vi "Simulated1.vi"() -> ()   [LabVIEW 2011]
doc: "This VI demonstrates how to control a simulated Robotics Starter Kit 1.0 robot. With a few modifications, you can deploy this VI to the Single-Board RIO 9631 on a real robot, and it runs on the real-time controller. For more information about how to modify this VI so you can deploy it to real hardware, refer to the <B>Robotics Module>>Simulating Mobile Robots</B> book on the <B>Contents</B> tab of the LabVIEW Help."
uses:
  <vilib>/Platform/TimedLoop/XDataNode/XDataNode.xnode
  <vilib>/Platform/TimedLoop/XDataNode/nitl_modes.ctl
  <vilib>/Platform/TimedLoop/XDataNode/XDNodeRunTimeDep.lvlib
  <vilib>/Platform/TimedLoop/XDataNode/wakeup.ctl
  <vilib>/Platform/TimedLoop/XDataNode/timing_clust.ctl
  <vilib>/robotics/Starter Kit/1.0/Sim Host Interface/NI_Robotics_Starter Kit Host_Sim_1.0.lvclass
  <vilib>/robotics/Simulator/NI_Robotics_Simulator.lvlib
  <vilib>/Analysis/Matrix/NI_Matrix.lvlib
  <vilib>/robotics/Starter Kit/Host Interface/NI_Robotics_Starter Kit Host.lvclass
  <vilib>/Analysis/Matrix/Numeric/Conversions/Array To Matrix - RA.vi
  <vilib>/Analysis/Matrix/Datatypes/RealMatrix.ctl
panel:
  out "Zigmar":dbl[](array[numeric])
  out "Zigma":dbl[](array[numeric])
  out "Xr-X":dbl[](array[numeric])
  out "Error":T1
  out "XY Graph":cluster{dbl[], dbl[]}(graph)
  in  "Kp W":dbl step=0.01
  in  "Kp VL":dbl step=0.01
  out "Numeric":i32
  in  "Paso":dbl
  in  "Tiempo":dbl
  in  "stop":bool
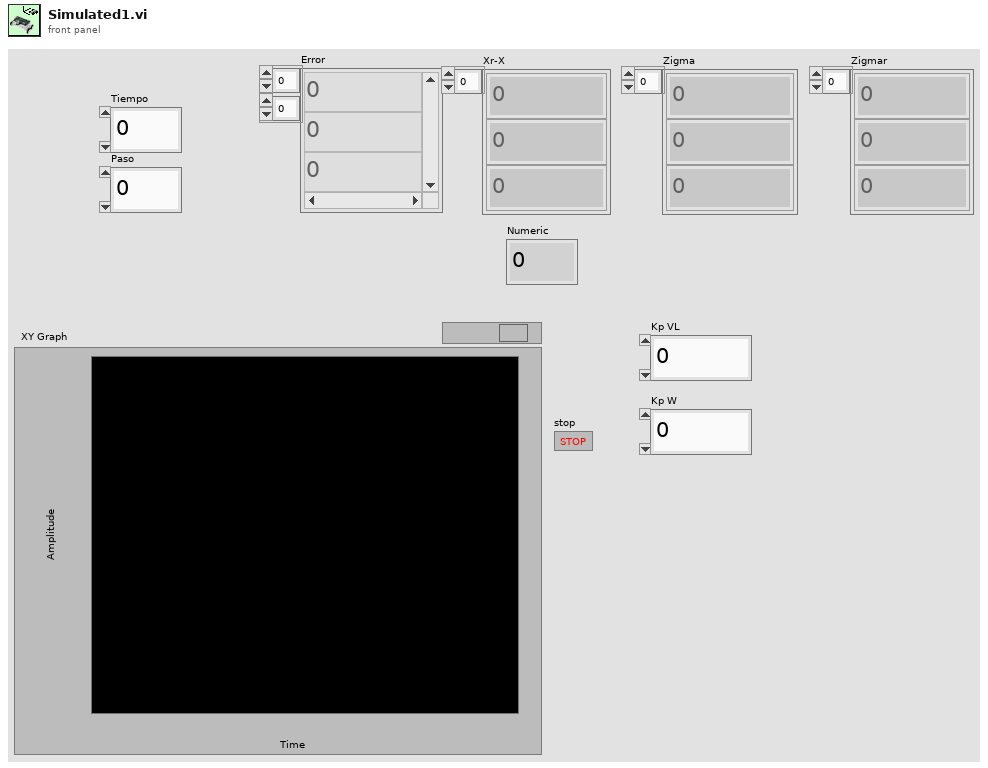
[diagram p1: front panel]
types:
  T1 = typedef "NI_Matrix.lvlib/RealMatrix.ctl" = dbl[][]
  T2 = typedef "XDNodeRunTimeDep.lvlib/timing_clust.ctl" = cluster{"Expected End [f-1]":u64, "Actual End [f-1]":u64, "Finished Late? [f-1]":bool, "Expected End [i-1]":u64, "Actual End [i-1]":u64, "Finished Late? [i-1]":bool, "Expected Start [i]":u64, "Actual Start [i]":u64, "Expected Start [f]":u64, "Actual Start [f]":u64, "Source Name":string, "Structure Name":string, "Period":i64, "Deadline":i64, "Offset":i64, "Start":i64, "Priority":i32, "Timeout":i32, "Mode":T3, "Wakeup Reason":T4, "Error":errorcluster, "Source Type":string, "Secondary Source Type":string, "Global End Time":u64, "Global Start Time":u64, "Frame Duration":u64, "Iteration Duration":u64, "Assigned CPU":i32, "I/O Scan Engine Mode":u32}
  T3 = typedef "XDNodeRunTimeDep.lvlib/nitl_modes.ctl" = enum32{"No Change", "Process missed periods, maintain original phase", "Discard missed periods, maintain original phase", "Process missed periods, ignore original phase", "Discard missed periods, ignore original phase"}
  T4 = typedef "XDNodeRunTimeDep.lvlib/wakeup.ctl" = enum32{"Normal", "Aborted", "Asynchronous wakeup", "Timing source error", "Timed loop error", "Timeout"}
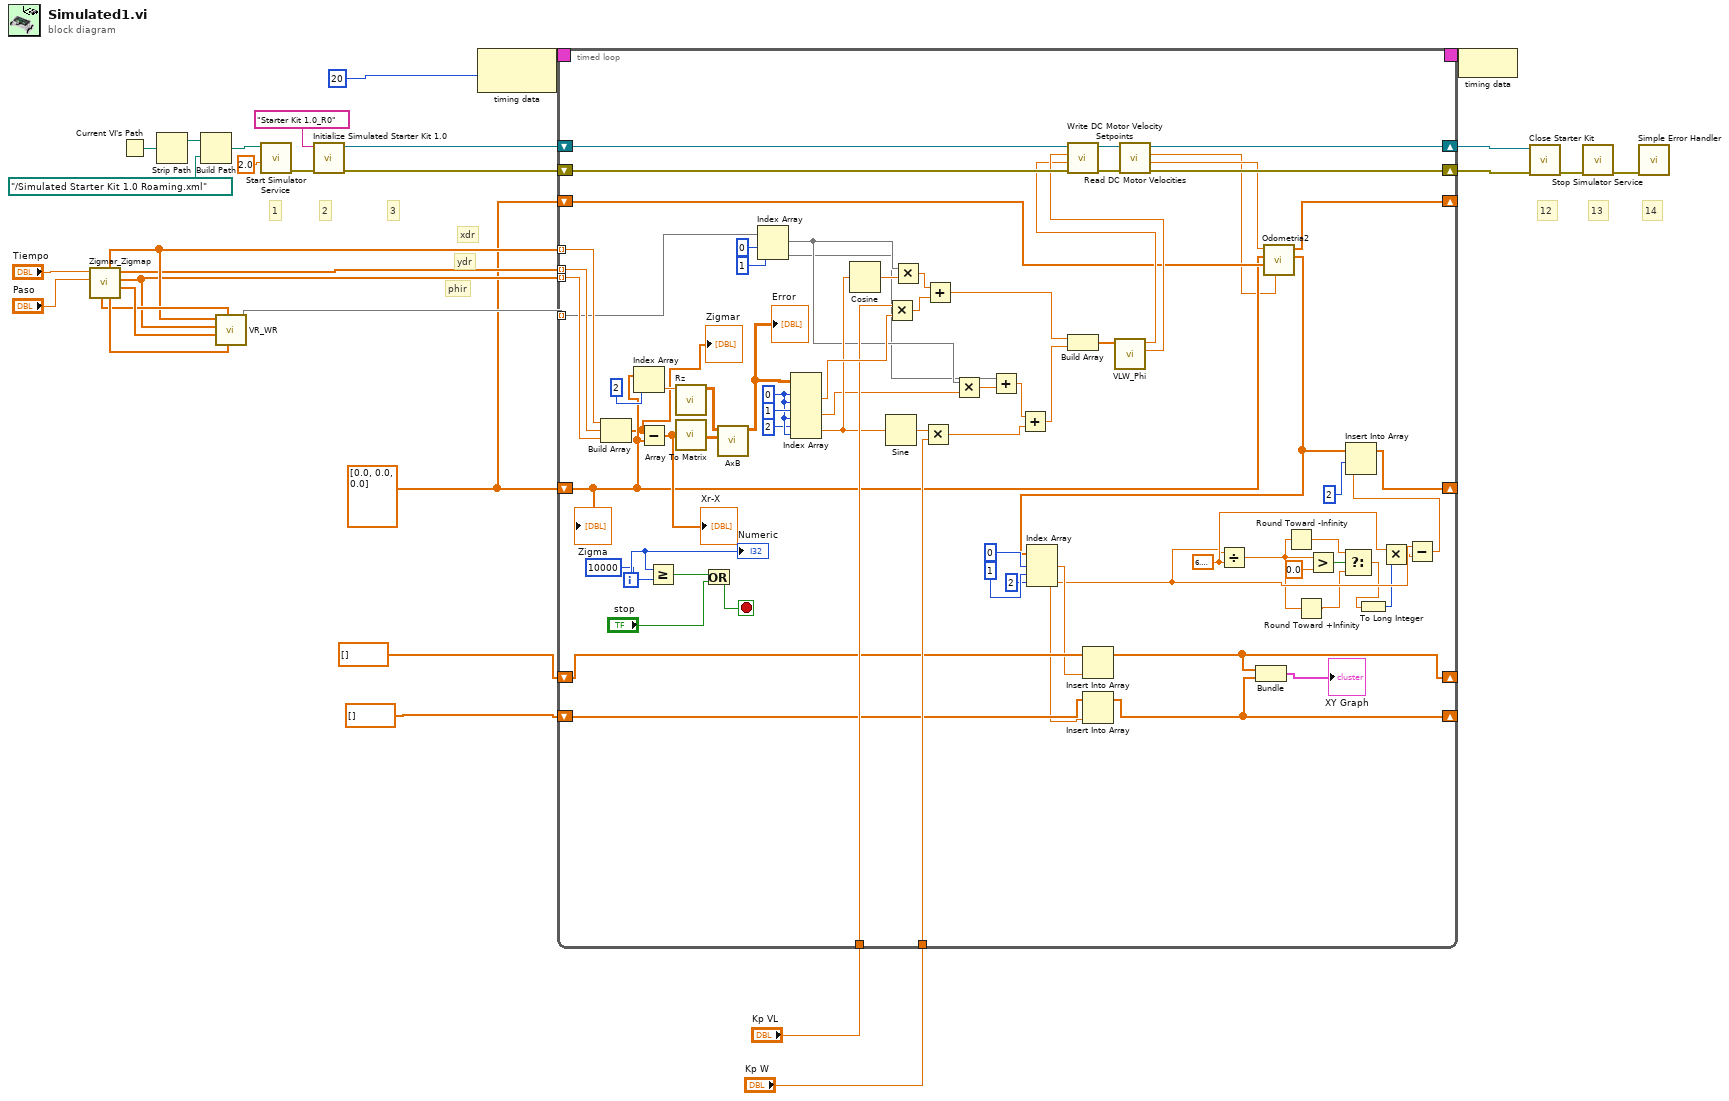
[diagram p0: block diagram]
diagram:
  w3 = dbl[] [0.0, 0.0, 0.0]
  # "phir"
  # "ydr"
  # "xdr"
  # "14"
  # "13"
  # "12"
  # "3"
  # "2"
  # "1"
  n1 = call "Zigmar_Zigmap.vi"("Paso"="Paso", "Tiempo"="Tiempo") -> ("Xdrp"=w11:dbl[], "Phir"=w6:dbl[], "Ydr"=w7:dbl[], "Ydrp"=w12:dbl[], "Xdr"=w8:dbl[], "Phirp"=w10:dbl[])  [unwired: 4 in]
  n2 = Current VI's Path() -> (path=w29:path)
  n3 = Strip Path(path=w29) -> (stripped path=w30:path)  [unwired: 1 out]
  n4 = Build Path(base path=w30, name or relative path=path "../Simulated Starter Kit 1.0 Roaming.xml" ("Simulation Manifest File")) -> (appended path=w20:path)
  n5 = call "VR_WR.vi"("Ydrp"=w12, "Phirp"=w10, "Xdrp"=w11, "Phir"=w6, 11:w8) -> (3:w9)  [unwired: 6 in]
  n6 = call <vilib>:"Start Simulator Service.vi"("step size (ms)"=2.0, "manifest file"=w20) -> ("error out"=w18:errorcluster)  [unwired: 9 in]
  n7 = call <vilib>:"Initialize Simulated Starter Kit 1.0.vi"("error in (no error)"=w18, "robot ID"="Starter Kit 1.0_R0") -> ("error out"=w15:errorcluster, "simulated starter kit host 1.0 out"=w25:refnum<class "NI_Robotics_Starter Kit Host_Sim_1.0.lvclass">)  [unwired: 8 in]
  n8 = node-c288(i64 20 ("Period")) -> (w28:T2)
  n9 = timed-loop {
    shift-right: [w68] -> w24
    shift-left: w25 -> [w70]
    shift-right: [w67] -> w23
    shift-left: w15 -> [w69]
    timing: w28 -> [_]
    timing-out: [_] -> w27
    tunnel: w9 -> [w93] mode=indexing
    tunnel: w8 -> [w105] mode=indexing
    tunnel: w7 -> [w104] mode=indexing
    tunnel: w6 -> [w103] mode=indexing
    shift-right: [w41] -> _
    shift-left: w3 -> [w59]
    tunnel: "Kp VL" -> [w88]
    tunnel: "Kp W" -> [w82]
    shift-right: [w60] -> _
    shift-left: w3 -> [w61]
    shift-right: [w52] -> _
    shift-left: dbl[] [] -> [w58]
    shift-right: [w51] -> _
    shift-left: dbl[] [] -> [w54]
    i -> [w64]
    stop <- w100 stop-if-true
    w44 = 6.283185307179586
    w91 = 0 ("index (row)")
    n10 = Build Array(w105, w104, w103) -> (w46:dbl[])
    "Zigmar" <- w46
    n11 = Index Array(array=w59, index=2) -> (element=w102:dbl)
    n12 = Subtract(x=w46, y=w59) -> (x-y=w97:dbl[])
    "Xr-X" <- w97
    n13 = Greater Or Equal?(x=w64, y=10000 ("x")) -> (x >= y?=w62:bool)
    n14 = call "Rz.vi"("theta"=w102) -> ("RotacionalZ"=w98:T1)  [unwired: 10 in]
    n15 = call-poly <vilib>:"Array To Matrix.vi"("Real 1D Array"=w97) -> ("Real Matrix (Column Vector)"=w96:T1)
    n16 = Or(x=w62, y="stop") -> (x .or. y?=w100:bool)
    n17 = call "AxB.vi"("B"=w96, "A"=w98) -> ("AxB"=w47:T1)  [unwired: 9 in]
    "Error" <- w47
    n18 = Index Array(array=w93, index #1=0 ("index"), index #2=1 ("index")) -> (element #1=w77, element #2=w76)
    n19 = Index Array(array=w47, index (row) #1=w91, index (col) #1=w91, index (row) #2=1 ("index (row)"), index (col) #2=w91, index (row) #3=2 ("index (row)"), index (col) #3=w91) -> (element #1=w89:dbl, element #2=w78:dbl, element #3=w84:dbl)
    n20 = Cosine(x=w84) -> (cos(x)=w87:dbl)
    n21 = Sine(x=w84) -> (sin(x)=w83:dbl)
    n22 = Multiply(x=w88, y=w89) -> (x*y=w86:dbl)
    n23 = Multiply(x=w77, y=w87) -> (x*y=w85:dbl)
    n24 = Multiply(x=w83, y=w82) -> (x*y=w79:dbl)
    n25 = Add(x=w85, y=w86) -> (x+y=w74:dbl)
    n26 = Multiply(x=w77, y=w78) -> (x*y=w81:dbl)
    n27 = Add(x=w76, y=w81) -> (x+y=w80:dbl)
    n28 = Add(x=w80, y=w79) -> (x+y=w73:dbl)
    n29 = Build Array(w74, w73) -> (w75:dbl[])
    n30 = call "VLW_Phi.vi"("VL/W"=w75) -> ("PhiL"=w66:dbl, "PhiR"=w65:dbl)  [unwired: 9 in]
    n31 = call <vilib>:"Write DC Motor Velocity Setpoints.vi"("error in (no error)"=w69, "right motor ccw velocity (rad/s)"=w65, "left motor ccw velocity (rad/s)"=w66, "starter kit host in"=w70) -> ("error out"=w72:errorcluster, "starter kit host out"=w71:refnum<class "NI_Robotics_Starter Kit Host_Sim_1.0.lvclass">)  [unwired: 6 in]
    n32 = call <vilib>:"Read DC Motor Velocities.vi"("error in (no error)"=w72, "starter kit host in"=w71) -> ("error out"=w67:errorcluster, "right motor ccw velocity (rad/s)"=w49:dbl, "left motor ccw velocity (rad/s)"=w48:dbl, "starter kit host out"=w68:refnum<class "NI_Robotics_Starter Kit Host_Sim_1.0.lvclass">)  [unwired: 6 in]
    n33 = call "Odometria2.vi"("left motor ccw velocity (rad/s)"=w48, "Arrastrado"=w61, "Zigma"=w59, "right motor ccw velocity (rad/s)"=w49) -> ("Array out"=w42:dbl[], "Arrastrad_out"=w60:dbl[])  [unwired: 6 in]
    n34 = Index Array(array=w42, index #1=0 ("index"), index #2=1 ("index"), index #3=2 ("index")) -> (element #1=w55:dbl, element #2=w53:dbl, element #3=w39:dbl)
    n35 = Insert Into Array(array=w58, new element=w55) -> (w52:dbl[])  [unwired: 1 in]
    n36 = Insert Into Array(array=w54, new element=w53) -> (w51:dbl[])  [unwired: 1 in]
    n37 = Divide(x=w39, y=w44) -> (x/y=w34:dbl)
    n38 = Bundle(w52, w51) -> (→"XY Graph":cluster{dbl[], dbl[]})  [unwired: 1 in]
    n39 = Round Toward -Infinity(1:w34) -> (0:w36:dbl)
    n40 = Round Toward +Infinity(x=w34) -> (ceil(x): smallest int >= x=w33:dbl)
    n41 = Greater?(x=w34, y=0.0) -> (0:w38:bool)
    n42 = Select(t=w36, s=w38, f=w33) -> (s? t:f=w31:dbl)
    n43 = To Long Integer(number=w31) -> (32bit integer=w32:i32)
    n44 = Multiply(x=w44, y=w32) -> (x*y=w37:dbl)
    n45 = Subtract(x=w39, y=w37) -> (x-y=w43:dbl)
    n46 = Insert Into Array(array=w42, index=2, new element=w43) -> (w41:dbl[])
    "Numeric" <- w64
    "Zigma" <- w59
  }
  n47 = node-c288(w27) -> ()
  n48 = call-dynamic "Close Starter Kit.vi"("error in (no error)"=w23, "starter kit host in"=w24) -> ("error out"=w17:errorcluster)  [unwired: 9 in]
  n49 = call <vilib>:"Stop Simulator Service.vi"("error in (no error)"=w17) -> ("error out"=w16:errorcluster)  [unwired: 10 in]
  n50 = call <vilib>:"Simple Error Handler.vi"("error in (no error)"=w16) -> ()  [unwired: 4 in, 5 out]
